vi "login simple.vi"() -> (3 "pass - fail":bool)   [LabVIEW 2019]
panel:
  in  "cancel":bool
  out "Type password!    checking....":i32(slide) scale=0.0..20.0
  in  "psw":string
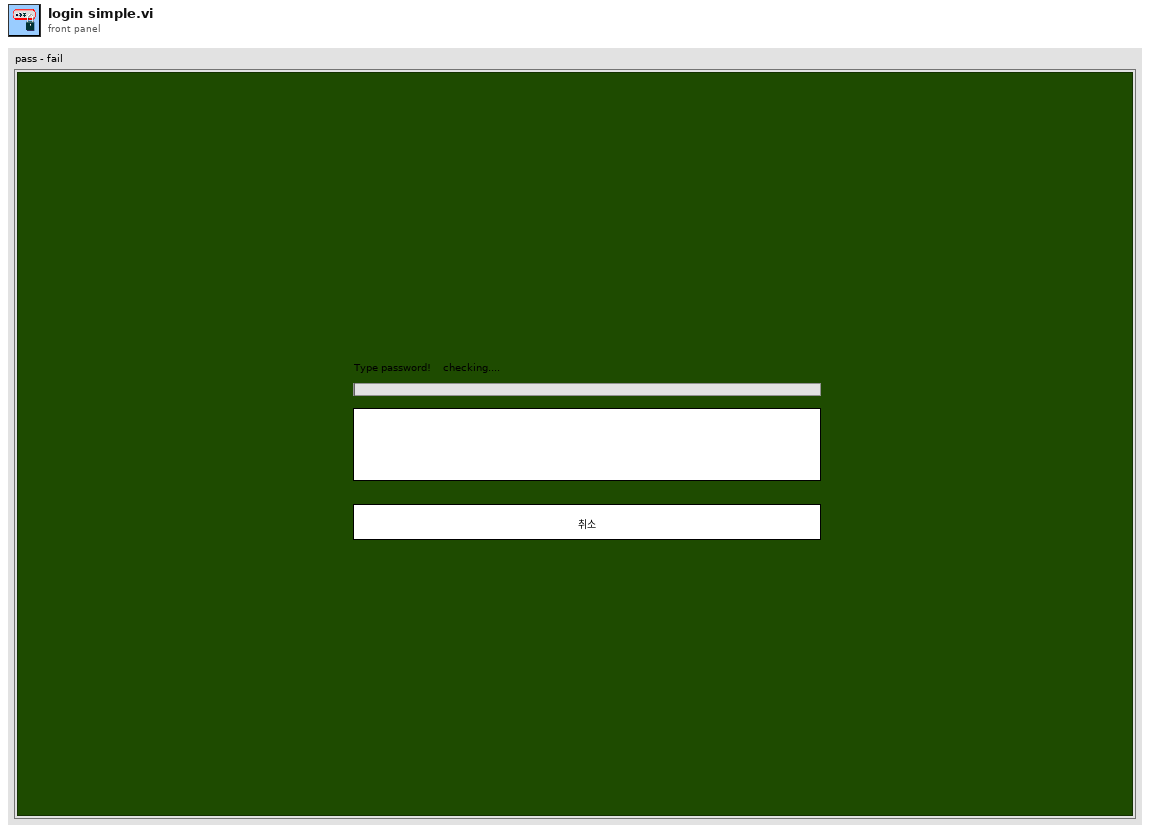
[diagram p1: front panel]
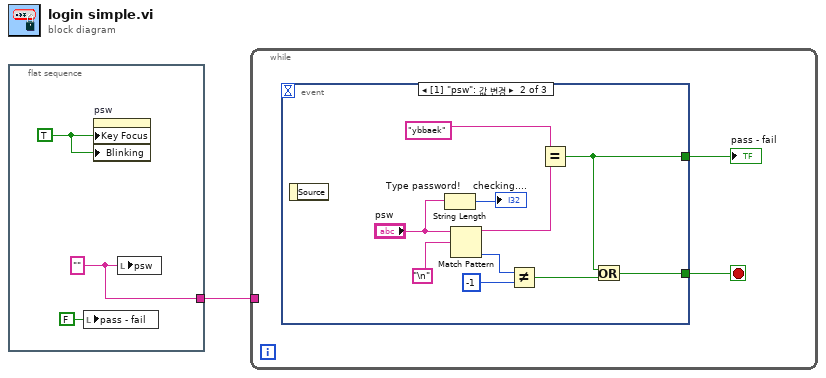
[diagram p0: block diagram]
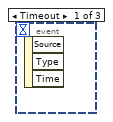
[diagram p2: hidden frame]
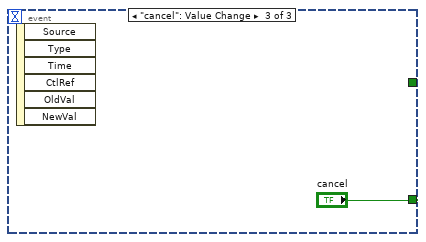
[diagram p3: hidden frame]
diagram:
  n1 = flat-sequence {
    tunnel: [w4] -> w1
    frame #0 {
      w2 = TRUE ("키 포커스")
      w4 = "" ("psw")
      n2 = local write "pass - fail"(FALSE ("pass - fail")) -> ()
      n3 = property on="psw" class="Str"("Key Focus"=w2, "Blinking"=w2) -> ()  [unwired: 2 in, 2 out]
      n4 = local write "psw"(w4) -> ()
    }
  }
  n5 = while {
    tunnel: w1 -> [_]
    stop <- w6 stop-if-true
    n6 = event shown="[1] \"psw\": 값 변경" {
      selector: _ -> [_ _ _]
      dyn-events: _ -> [_ _ _]
      timeout: _ -> [_ _ _]
      tunnel: [_ w7 "cancel"] -> w6
      tunnel: [_ w8 _] -> w5
      event Timeout {
        n7 = event-data() -> ()  [unwired: 1 in, 3 out]
      }
      event "psw": Value Change {
        n8 = event-data() -> ()  [unwired: 1 in, 1 out]
        n9 = String Length(string="psw") -> (length=→"Type password!    checking....":i32)
        n10 = Match Pattern(string="psw", regular expression="\n") -> (before substring=w10:string, offset past match=w14:i32)  [unwired: 1 in, 2 out]
        n11 = Not Equal?(x=w14, y=-1) -> (x != y?=w9:bool)
        n12 = Equal?(x="ybbaek", y=w10) -> (x = y?=w8:bool)
        n13 = Or(x=w8, y=w9) -> (x .or. y?=w7:bool)
      }
      event "cancel": Value Change {
        n14 = event-data() -> ()  [unwired: 1 in, 6 out]
      }
    }
    "pass - fail" <- w5
  }
